vi "Triangulation Function.vi"(9 "output selector":T1, 10 "data":T2, 11 "X":dbl[](array[numeric])) -> (0 "error out":errorcluster, 1 "inequality constraint function values":dbl[](array[numeric]), 2 "equality constraint function values":dbl[](array[numeric]), 3 "objective function value":dbl)   [LabVIEW 2012]
doc: "This template is the starting point for creating an objective function, equality constraint function and inequality constraint function to be passed to the Constrained Nonlinear Optimization.vi."
uses:
  <vilib>/gmath/NumericalOptimization/objective function data.ctl
  <vilib>/gmath/NumericalOptimization/cno_output select.ctl
  <vilib>/gmath/NI_Gmath.lvlib
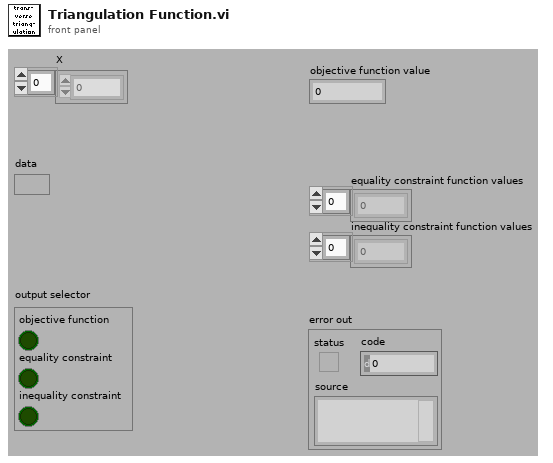
[diagram p1: front panel]
types:
  T1 = typedef "NI_Gmath.lvlib/cno_output select.ctl" = cluster{"objective function":bool, "equality constraint":bool, "inequality constraint":bool}
  T2 = typedef "NI_Gmath.lvlib/objective function data.ctl" = variant
  T3 = cluster{"x_prime":dbl, "y_prime":dbl, "z_prime":dbl}
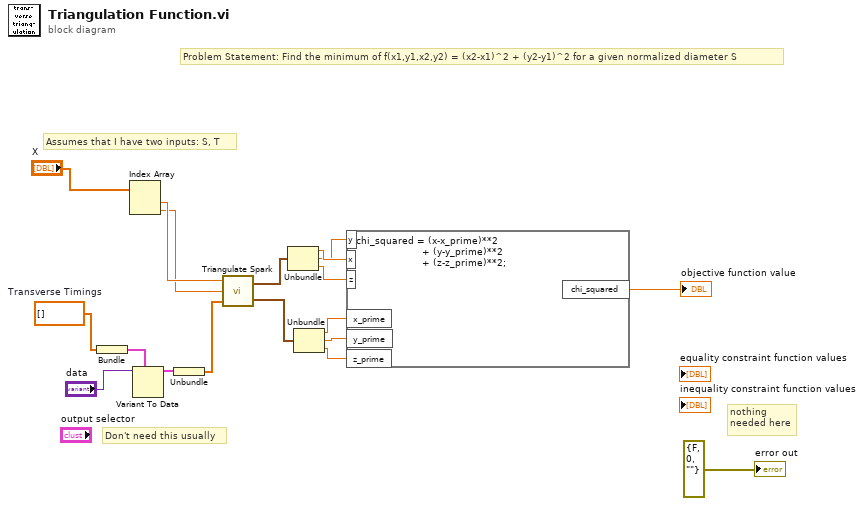
[diagram p0: block diagram]
diagram:
  w16 = dbl[] []  # Transverse Timings
  # "nothing \nneeded here"
  # "Problem Statement: Find the minimum of f(x1,y1,x2,y2) = (x2-x1)^2 + (y2-y1)^2 for a given normalized diameter S"
  # "Don't need this usually"
  # "Assumes that I have two inputs: S, T"
  n1 = Bundle("Transverse Timings"=w16) -> (w14:cluster{"Transverse Timings":dbl[]})  [unwired: 1 in]
  n2 = Index Array(array="X") -> (element #1=w11:dbl, element #2=w10:dbl)  [unwired: 2 in]
  n3 = Variant To Data(type=w14, Variant="data") -> (data=w13:cluster{"Transverse Timings":dbl[]})  [unwired: 1 in, 1 out]
  n4 = Unbundle(w13) -> ("Transverse Timings"=w9:dbl[])
  n5 = call <userlib>:"Triangulate Spark.vi"("timings"=w9, "cavity length (s)"=w10, "cavity diameter (s)"=w11) -> ("coordinates_prime"=w7:T3, "coordinates"=w8:cluster{"x":dbl, "y":dbl, "z":dbl})  [unwired: 1 in]
  n6 = Unbundle(w8) -> ("x"=w6:dbl, "y"=w5:dbl, "z"=w4:dbl)
  n7 = Unbundle(w7) -> ("x_prime"=w3:dbl, "y_prime"=w2:dbl, "z_prime"=w1:dbl)
  n8 = formula code="chi_squared = (x-x_prime)**2\n                      + (y-y_prime)**2\n                      + (z-z_prime)**2;"("x"=w6, "y"=w5, "z"=w4, "x_prime"=w3, "y_prime"=w2, "z_prime"=w1) -> ("chi_squared"=→"objective function value":dbl)
  "error out" <- errorcluster {"status"=FALSE, "code"=0, "source"=""} ("error out")
